vi "RS_SMBV100A_NMEA0183_close.vi"(7 "error in":errorcluster, 10 "NMEA0183 Ref":refnum<k7>) -> (0 "error out":errorcluster)   [LabVIEW 2018]
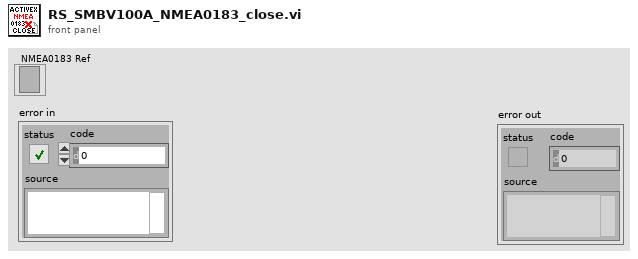
[diagram p1: front panel]
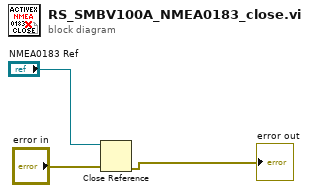
[diagram p0: block diagram]
diagram:
  n1 = Close Reference(reference="NMEA0183 Ref", error in (no error)="error in") -> (error out=→"error out":errorcluster)
